vi "dosimat_write_command.vi"(3 "error in":errorcluster, 4 "write buffer":string, 5 "Dosimat Port In":refnum<visa-resource-name>="COM1") -> (0 "error out":errorcluster, 1 "read buffer":string, 2 "Dosimat Port Out":refnum<visa-resource-name>="COM1")   [LabVIEW 2010]
panel:
  # "mooseNote: tell it which of the commands \nto write and it will send it to the 876"
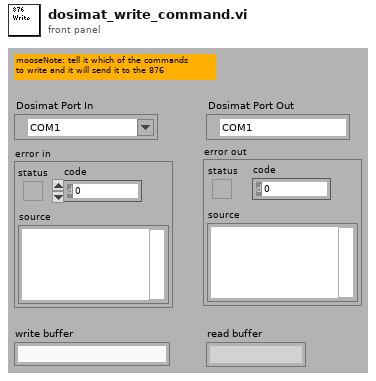
[diagram p1: front panel]
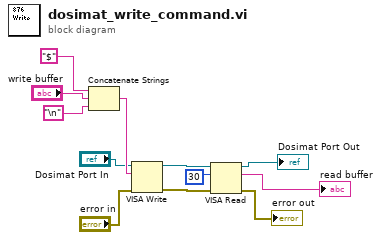
[diagram p0: block diagram]
diagram:
  n1 = Concatenate Strings("$" ("string"), "write buffer", "\n") -> (w7:string)
  n2 = VISA Write(VISA resource name="Dosimat Port In", write buffer=w7, error in (no error)="error in") -> (VISA resource name out=w12:refnum<visa-resource-name>, error out=w11:errorcluster)  [unwired: 1 out]
  n3 = VISA Read(VISA resource name=w12, byte count=u32 30, error in (no error)=w11) -> (VISA resource name out=→"Dosimat Port Out":refnum<visa-resource-name>, read buffer=→"read buffer":string, error out=→"error out":errorcluster)  [unwired: 1 out]
